vi "CollectorWrap.vi"(7 "Action":T1=enum."Collect", 8 "error in":errorcluster) -> (0 "error out":errorcluster)   [LabVIEW 2013]
uses:
  CollectorWrapAction.ctl
  DoubleSolenoidAction.ctl
  RollerAction.ctl
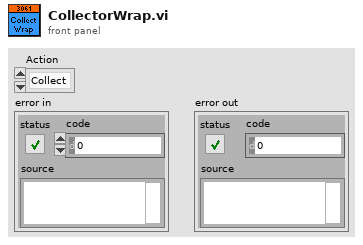
[diagram p1: front panel]
types:
  T1 = typedef "CollectorWrapAction.ctl" = enum16{"PreCollect", "Collect", "Stop"}
  T2 = typedef "DoubleSolenoidAction.ctl" = enum16{"Init", "Middle", "In", "Out"}
  T3 = typedef "RollerAction.ctl" = enum16{"Init", "Off", "Forward", "Reverse"}
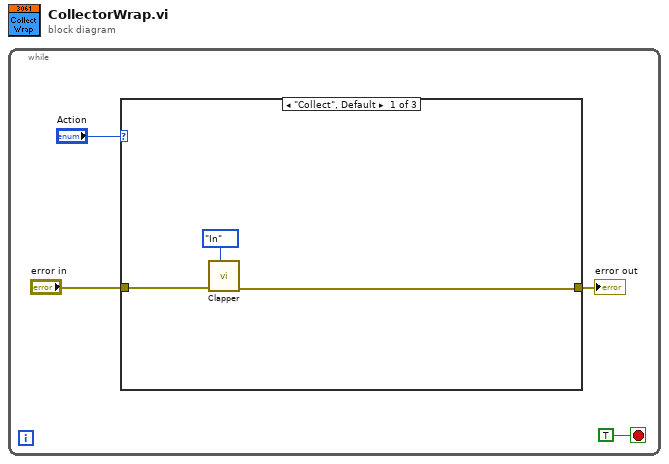
[diagram p0: block diagram]
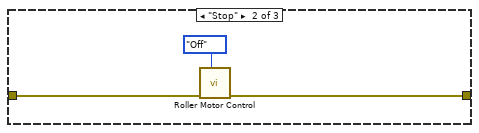
[diagram p2: hidden frame]
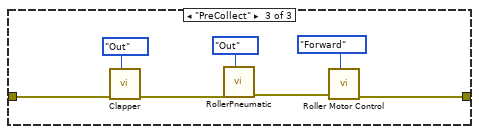
[diagram p3: hidden frame]
diagram:
  n1 = while {
    stop <- TRUE stop-if-true
    n2 = case shown="\"Collect\", Default" "Action" {
      tunnel: "error in" -> [w7 w10 w15]
      tunnel: [w6 w9 w17] -> w1
      frame "Collect", Default {
        n3 = call "Clapper.vi"("State"=DoubleSolenoidAction."In", "Error in"=w7) -> ("Error out"=w6:errorcluster)  [unwired: 9 in]
      }
      frame "Stop" {
        n4 = call "Roller Motor Control.vi"("Action"=RollerAction."Off", "Error in"=w10) -> ("Error out"=w9:errorcluster)  [unwired: 9 in]
      }
      frame "PreCollect" {
        n5 = call "Clapper.vi"("State"=DoubleSolenoidAction."Out", "Error in"=w15) -> ("Error out"=w14:errorcluster)  [unwired: 9 in]
        n6 = call "RollerPneumatic.vi"("State"=DoubleSolenoidAction."Out", "Error in"=w14) -> ("Error out"=w13:errorcluster)  [unwired: 9 in]
        n7 = call "Roller Motor Control.vi"("Action"=RollerAction."Forward", "Error in"=w13) -> ("Error out"=w17:errorcluster)  [unwired: 9 in]
      }
    }
    "error out" <- w1
  }
